vi "ADD TEST HEAD.vi"(4 "测试头文件.测试环境":string, 6 "dp/dt":string, 8 "pmax":string, 9 "ch no":i32, 11 "Temp in":T1={"Vibr Chn Name"=[], "Analysis Chn Number"=0, "Index Vibration Waveform"={"t0"=timestamp(0 s since 1904-01-01), "dt"=1.0, "Y"=[]}, "Report Infomation"={"Test Name"="", "Tester"="", "Tempre Chart"=refnum, "Apli-Fre"=refnum, "Phase-Fre"=refnum, "Raw Data"=refnum}, "Vibr Apli - Fre"=[], "Vibr Phase - Fre"=[], "Error"={"status"=FALSE, "code"=0, "source"=""}, "Read Chan Name"="", "Test Info"={"Test Name"="", "Tester"=""}, "test data"=[{"t0"=timestamp(0 s since 1904-01-01), "dt"=1.0, "Y"=[]}, {"t0"=timestamp(0 s since 1904-01-01), "dt"=1.0, "Y"=[]}, {"t0"=timestamp(0 s since 1904-01-01), "dt"=1.0, "Y"=[]}, {"t0"=timestamp(0 s since 1904-01-01), "dt"=0.001, "Y"=[]}], "测试头文件"={"ch"=[], "测试环境"=""}, "CAl VAlUE"={"max_t"=[], "max_V"=[], "start_t"=[], "start_V"=[], "distance"=[], "unit"=""}}) -> (3 "Temp out":T1={"Vibr Chn Name"=[], "Analysis Chn Number"=0, "Index Vibration Waveform"={"t0"=timestamp(0 s since 1904-01-01), "dt"=1.0, "Y"=[]}, "Report Infomation"={"Test Name"="", "Tester"="", "Tempre Chart"=refnum, "Apli-Fre"=refnum, "Phase-Fre"=refnum, "Raw Data"=refnum}, "Vibr Apli - Fre"=[], "Vibr Phase - Fre"=[], "Error"={"status"=FALSE, "code"=0, "source"=""}, "Read Chan Name"="", "Test Info"={"Test Name"="", "Tester"=""}, "test data"=[{"t0"=timestamp(0 s since 1904-01-01), "dt"=1.0, "Y"=[]}, {"t0"=timestamp(0 s since 1904-01-01), "dt"=1.0, "Y"=[]}, {"t0"=timestamp(0 s since 1904-01-01), "dt"=1.0, "Y"=[]}, {"t0"=timestamp(0 s since 1904-01-01), "dt"=0.001, "Y"=[]}], "测试头文件"={"ch"=[], "测试环境"=""}, "CAl VAlUE"={"max_t"=[], "max_V"=[], "start_t"=[], "start_V"=[], "distance"=[], "unit"=""}})   [LabVIEW 2011]
uses:
  Ctrls/ana data.ctl
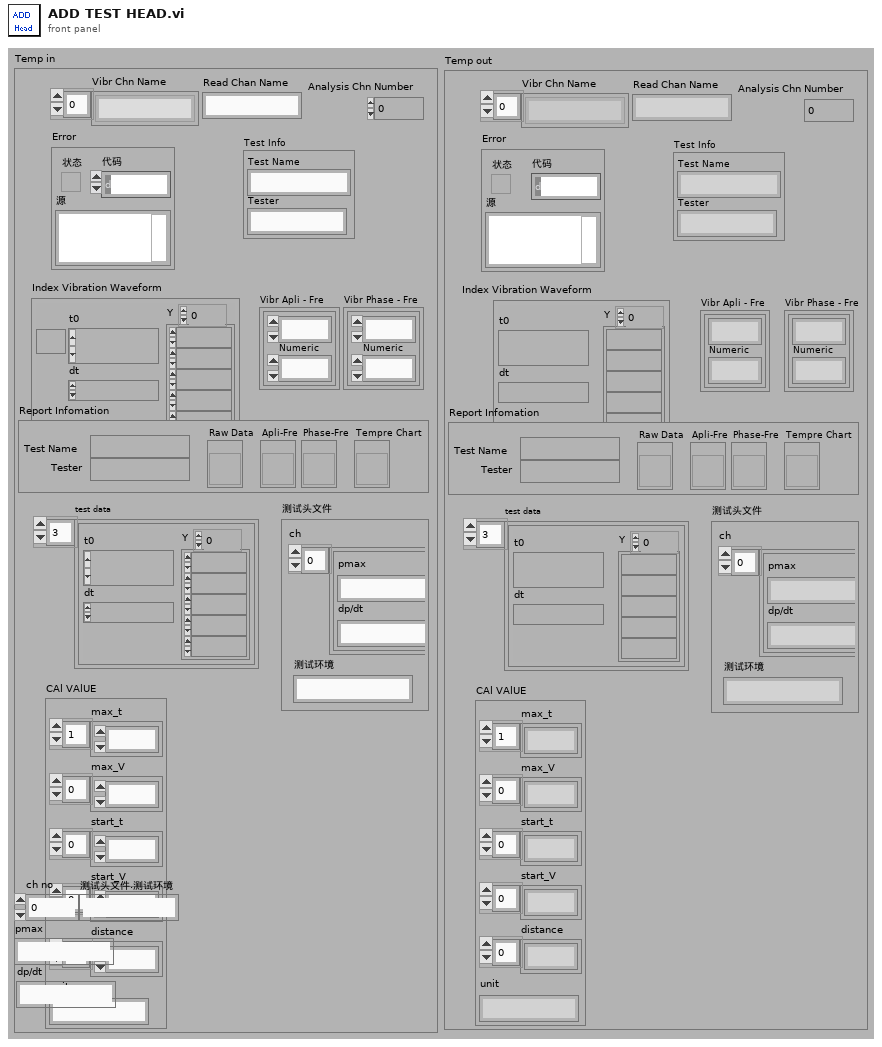
[diagram p1: front panel]
types:
  T1 = typedef "ana data.ctl" = cluster{"Vibr Chn Name":string[], "Analysis Chn Number":i32, "Index Vibration Waveform":waveform(dbl), "Report Infomation":cluster{"Test Name":string, "Tester":string, "Tempre Chart":refnum<vi>, "Apli-Fre":refnum<vi>, "Phase-Fre":refnum<vi>, "Raw Data":refnum<vi>}, "Vibr Apli - Fre":cluster{dbl, "Numeric":dbl}[], "Vibr Phase - Fre":cluster{dbl, "Numeric":dbl}[], "Error":errorcluster, "Read Chan Name":string, "Test Info":cluster{"Test Name":string, "Tester":string}, "test data":waveform(dbl)[], "测试头文件":cluster{"ch":cluster{"pmax":string, "dp/dt":string}[], "测试环境":string}, "CAl VAlUE":cluster{"max_t":dbl[], "max_V":dbl[], "start_t":dbl[], "start_V":dbl[], "distance":dbl[], "unit":string}}
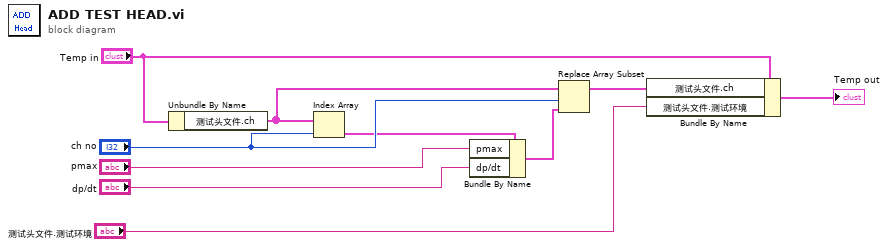
[diagram p0: block diagram]
diagram:
  n1 = Unbundle By Name("Temp in") -> ("测试头文件.ch"=w7:cluster{"pmax":string, "dp/dt":string}[])
  n2 = Index Array(array=w7, index="ch no") -> (element=w4:cluster{"pmax":string, "dp/dt":string})
  n3 = Bundle By Name(cluster=w4, "pmax"="pmax", "dp/dt"="dp/dt") -> (w3:cluster{"pmax":string, "dp/dt":string})
  n4 = Replace Array Subset(array=w7, new element=w3, index="ch no") -> (w6:cluster{"pmax":string, "dp/dt":string}[])
  n5 = Bundle By Name(cluster="Temp in", "测试头文件.ch"=w6, "测试头文件.测试环境"="测试头文件.测试环境") -> (→"Temp out":T1)
